vi "Auto Drive XY Right Automatic.vi"(0 "RobotDriveDevRef In":T2={"DevStatus"={"status"=FALSE, "code"=0, "source"=""}, "Motors[]"=[], "Square Inputs"=FALSE, "Max Output"=1.0}, 1 "Angle Offset":dbl, 3 "Movement":dbl=-1.0, 5 "Motor Output Range X":cluster{"output high":dbl, "output low":dbl}={"output high"=0.8, "output low"=-0.8}, 7 "PID Gains X":T1={"proportional gain (Kc)"=0.07, "integral time (Ti, min)"=0.0, "derivative time (Td, min)"=0.0}, 9 "Distance (in)":dbl=15.0 format="%#_13g", 11 "Time to Settle (ms)":u32=50, 12 "Min Time (ms)":u32=250, 13 "PID Gains Y":T1={"proportional gain (Kc)"=0.07, "integral time (Ti, min)"=0.0, "derivative time (Td, min)"=0.0}, 14 "Motor Output Range Y":cluster{"output high":dbl, "output low":dbl}={"output high"=0.7, "output low"=-0.7}, 15 "Max Time (ms)":u32=15000) -> (4 "RobotDriveDevRef Out":T2={"DevStatus"={"status"=FALSE, "code"=0, "source"=""}, "Motors[]"=[], "Square Inputs"=FALSE, "Max Output"=1.0})   [LabVIEW 2017]
uses:
  <vilib>/Rock Robotics/WPI/RobotDrive/WPI_RobotDriveDevRef.ctl
  <vilib>/Rock Robotics/WPI/MotorControl/WPI_MotorControlDeviceRef.ctl
  <vilib>/Rock Robotics/WPI/MotorControl/WPI_MotorControlType.ctl
  <vilib>/Rock Robotics/SystemInterfaces/DIO/FPGA_DIOPWMChannel.ctl
  <vilib>/Rock Robotics/WPI/PWM/WPI_PWMDeadband.ctl
  <vilib>/Rock Robotics/SystemInterfaces/DIO/FPGA_DIOChannel.ctl
  <vilib>/Rock Robotics/WPI/Solenoid/WPI_SolenoidValue.ctl
  Globals/Robot Global Data.vi
  <vilib>/addons/control/pid/pid.llb/PID (DBL).vi
  <vilib>/Rock Robotics/WPI/RobotDrive/WPI_RobotDriveArcadeDrive_Standard(NoSaturation).vi
  <vilib>/addons/control/pid/NI_PID_pid.lvlib
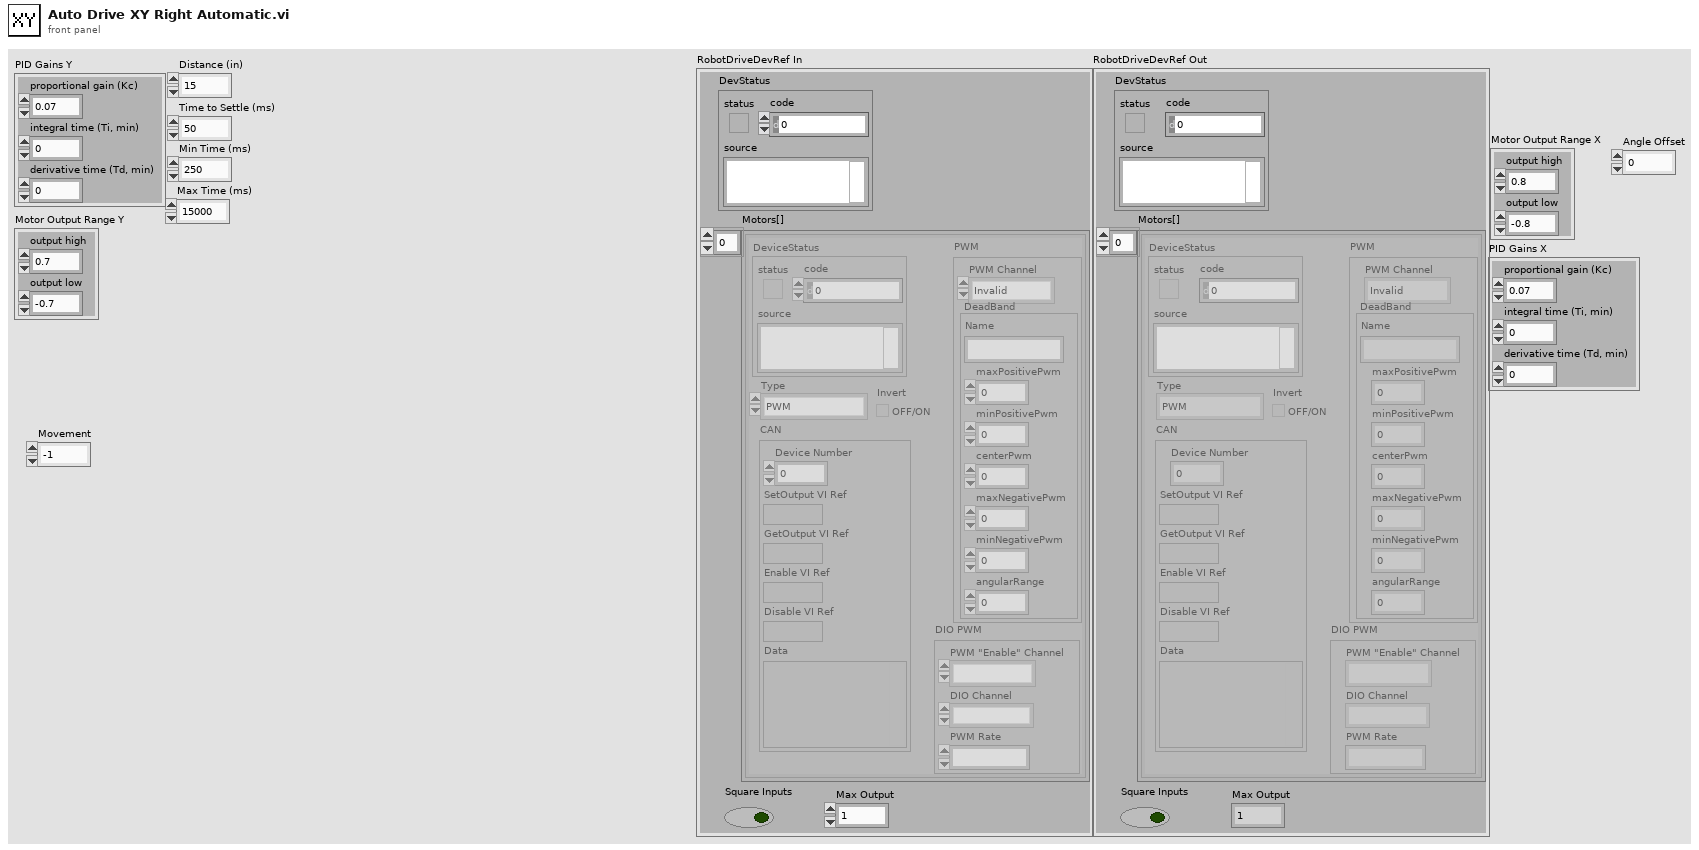
[diagram p1: front panel]
types:
  T1 = cluster{"proportional gain (Kc)":dbl, "integral time (Ti, min)":dbl, "derivative time (Td, min)":dbl}
  T2 = typedef "WPI_RobotDriveDevRef.ctl" = cluster{"DevStatus":errorcluster, "Motors[]":T3[], "Square Inputs":bool, "Max Output":dbl}
  T3 = typedef "WPI_MotorControlDeviceRef.ctl" = cluster{"DeviceStatus":errorcluster, "Type":T4, "PWM":cluster{"PWM Channel":T5, "DeadBand":T6}, "CAN":cluster{"Device Number":u8, "SetOutput VI Ref":variant, "GetOutput VI Ref":variant, "Enable VI Ref":variant, "Disable VI Ref":variant, "Data":variant}, "Invert":bool, "DIO PWM":cluster{"PWM \"Enable\" Channel":T5, "DIOChannel":T7, "PWM Rate":dbl}}
  T4 = typedef "WPI_MotorControlType.ctl" = enum16{"PWM", "CAN", "DIO PWM"}
  T5 = typedef "FPGA_DIOPWMChannel.ctl" = enum8{"PWM 0", "PWM 1", "PWM 2", "PWM 3", "PWM 4", "PWM 5", "PWM 6", "PWM 7", "PWM 8", "PWM 9", "PWM MXP 0", "PWM MXP 1", "PWM MXP 2", "PWM MXP 3", "PWM MXP 4", "PWM MXP 5", "PWM MXP 6", "PWM MXP 7", "PWM MXP 8", "PWM MXP 9", "Invalid"}
  T6 = typedef "WPI_PWMDeadband.ctl" = cluster{"Name":string, "maxPositivePwm":i32, "minPositivePwm":i32, "centerPwm":i32, "maxNegativePwm":i32, "minNegativePwm":i32, "angularRange":u16}
  T7 = typedef "FPGA_DIOChannel.ctl" = enum8{"DIO 0", "DIO 1", "DIO 2", "DIO 3", "DIO 4", "DIO 5", "DIO 6", "DIO 7", "DIO 8", "DIO 9", "DIO MXP 0", "DIO MXP 1", "DIO MXP 2", "DIO MXP 3", "DIO MXP 4", "DIO MXP 5", "DIO MXP 6", "DIO MXP 7", "DIO MXP 8", "DIO MXP 9", "DIO MXP 10", "DIO MXP 11", "DIO MXP 12", "DIO MXP 13", "DIO MXP 14", "DIO MXP 15", "SPI Port CS1", "SPI Port CS2", "SPI Port CS3", "SPI Port MISO", "SPI Port MOSI", "Invalid"}
  T8 = typedef "WPI_SolenoidValue.ctl" = enum16{"Off", "On", "Forward", "Reverse"}
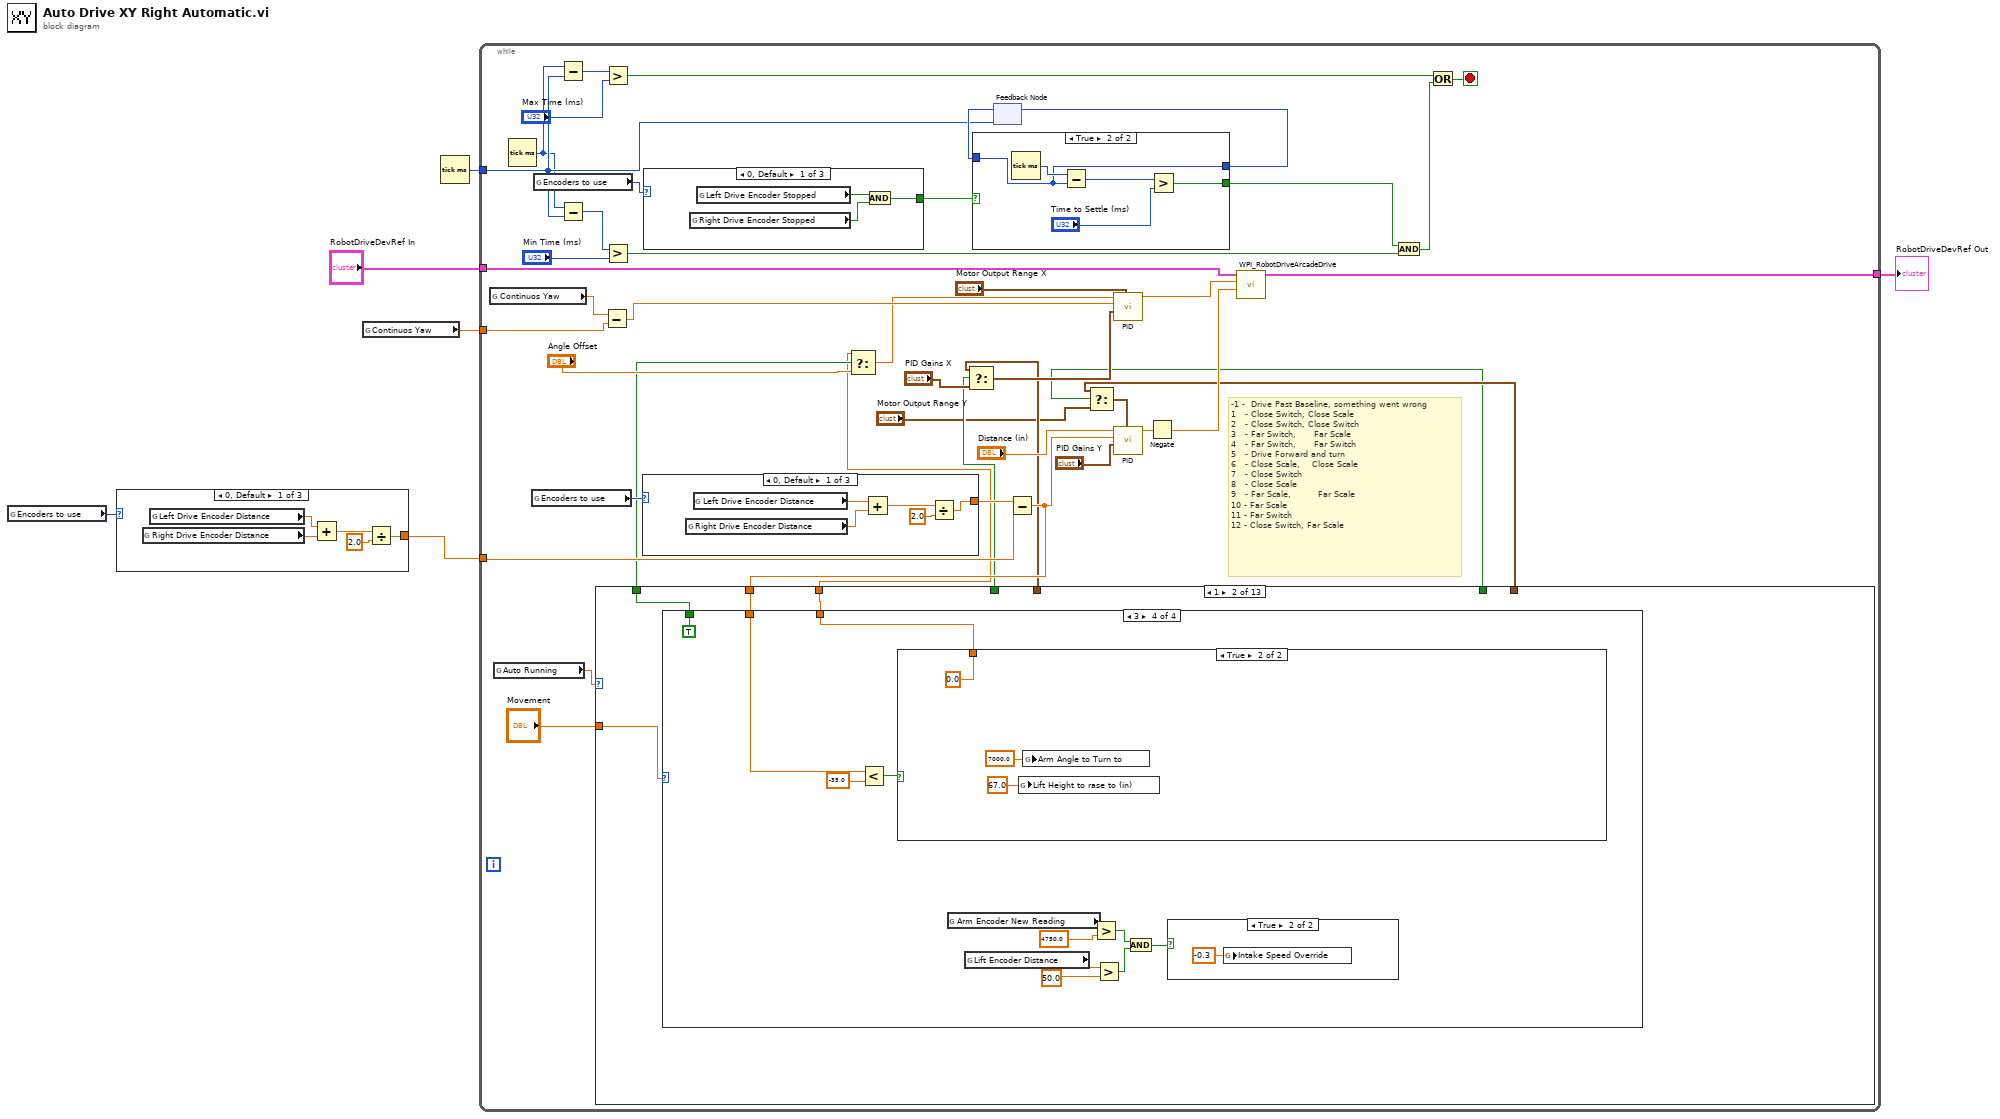
[diagram p0: block diagram]
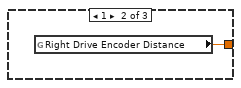
[diagram p2: hidden frame]
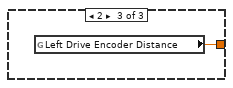
[diagram p3: hidden frame]
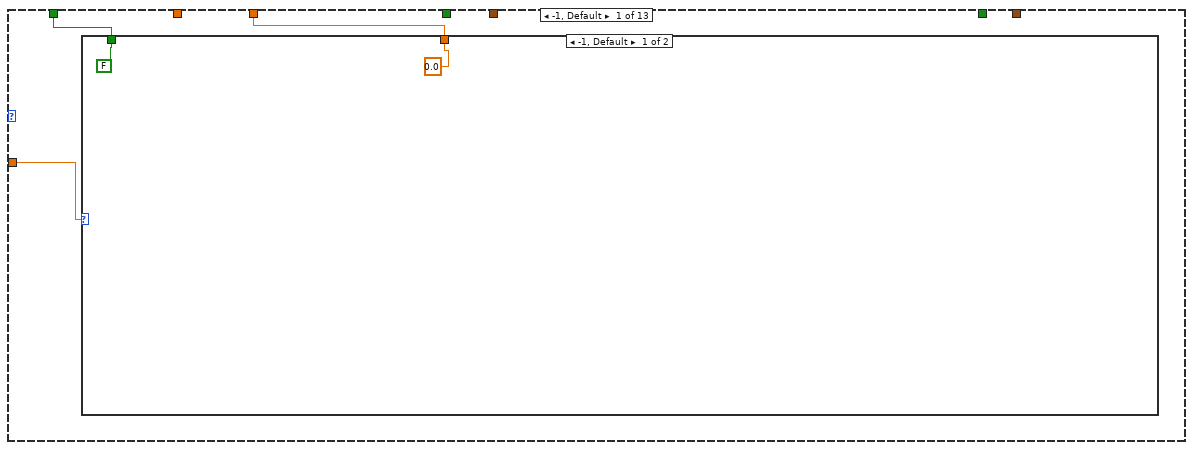
[diagram p4: hidden frame]
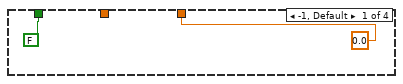
[diagram p6: hidden frame]
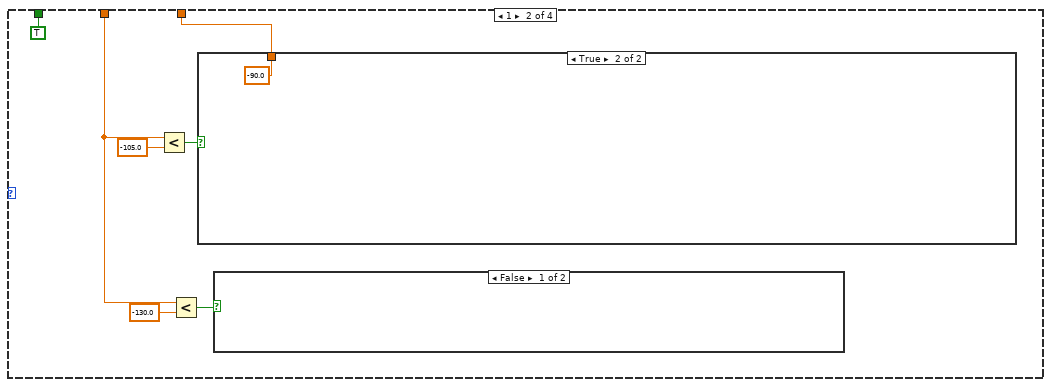
[diagram p7: hidden frame]
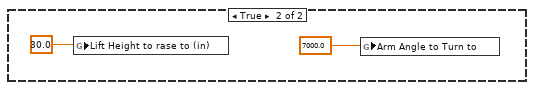
[diagram p8: hidden frame]
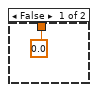
[diagram p9: hidden frame]
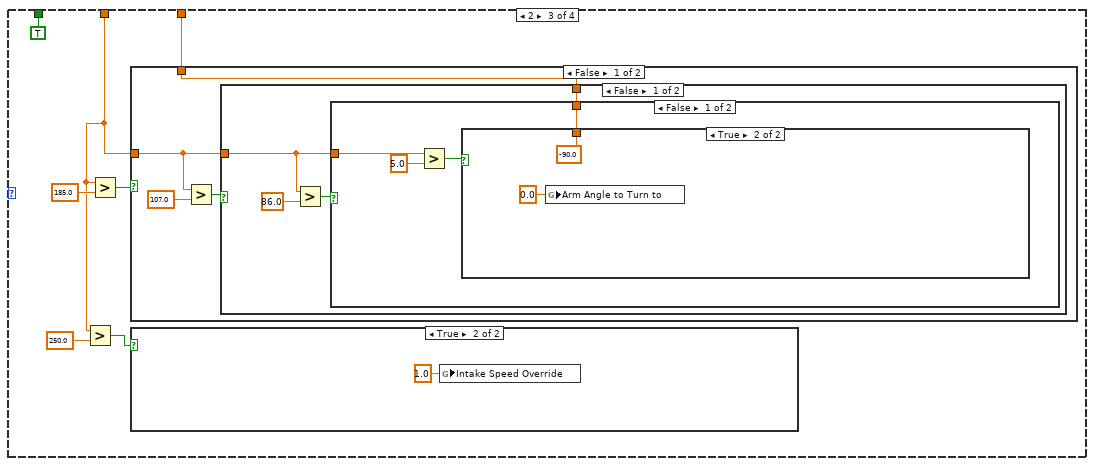
[diagram p10: hidden frame]
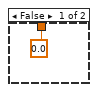
[diagram p11: hidden frame]
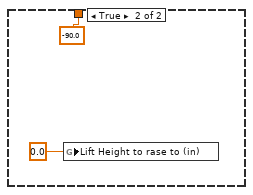
[diagram p12: hidden frame]
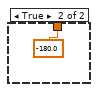
[diagram p13: hidden frame]
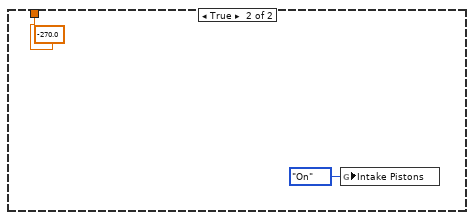
[diagram p14: hidden frame]
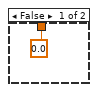
[diagram p17: hidden frame]
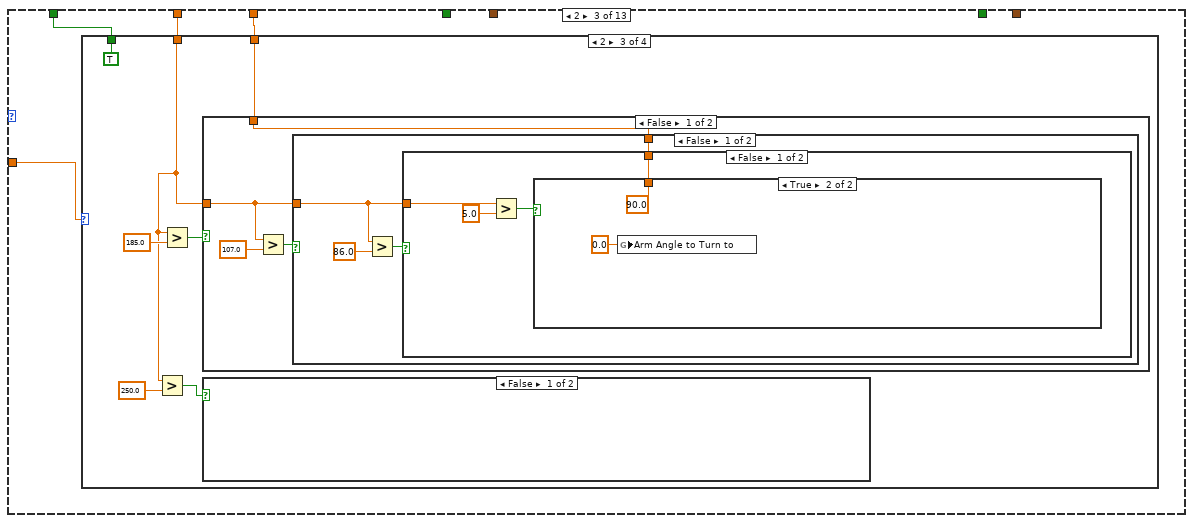
[diagram p18: hidden frame]
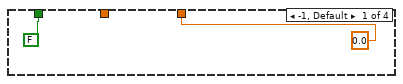
[diagram p19: hidden frame]
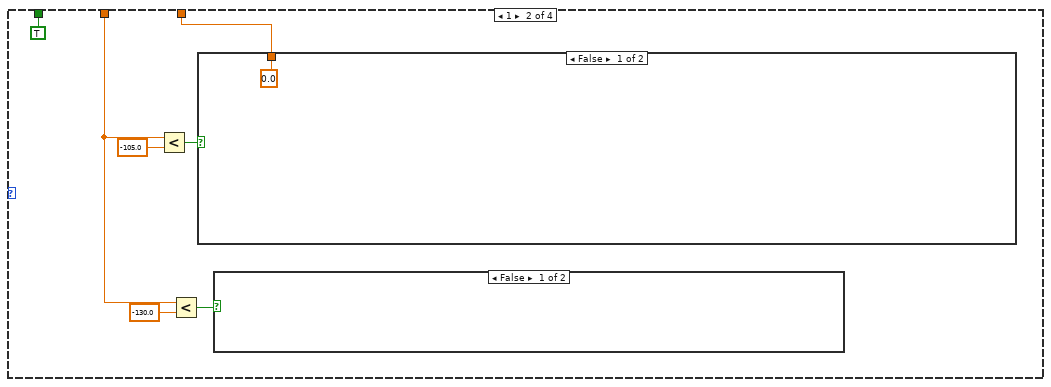
[diagram p20: hidden frame]
diagram:
  n1 = global read "Robot Global Data.vi" "Encoders to use"() -> (w2:u16)
  n2 = case shown="0, Default" w2 {
    tunnel: [w7 w12 w13] -> w6
    frame 0, Default {
      n3 = global read "Robot Global Data.vi" "Right Drive Encoder Distance"() -> (w10:dbl)
      n4 = global read "Robot Global Data.vi" "Left Drive Encoder Distance"() -> (w11:dbl)
      n5 = Add(x=w11, y=w10) -> (x+y=w9:dbl)
      n6 = Divide(x=w9, y=2.0) -> (x/y=w7:dbl)
    }
    frame 1 {
      n7 = global read "Robot Global Data.vi" "Right Drive Encoder Distance"() -> (w12:dbl)
    }
    frame 2 {
      n8 = global read "Robot Global Data.vi" "Left Drive Encoder Distance"() -> (w13:dbl)
    }
  }
  n9 = global read "Robot Global Data.vi" "Continuos Yaw"() -> (w1:dbl)
  n10 = Tick Count (ms)() -> (millisecond timer value=w5:u32)
  n11 = while {
    tunnel: "RobotDriveDevRef In" -> [w55]
    tunnel: w6 -> [w50]
    tunnel: w5 -> [w39]
    tunnel: [w49] -> w4
    tunnel: w1 -> [w30]
    stop <- w42 stop-if-true
    # "-1 -  Drive Past Baseline, something went wrong\n1   - Close Switch, Close Scale\n2   - Close Switch, Close Switch\n3   - Far Switch,      Far Scale\n4   - Far Switch,      Far Switch\n5   - Drive Forward and turn\n6   - Close Scale,    Close Scale\n7   - Close Switch\n8   - Close Scale\n9   - Far Scale,         Far Scale\n10 - Far Scale\n11 - Far Switch\n12 - Close Switch, Far Scale"
    n12 = global read "Robot Global Data.vi" "Continuos Yaw"() -> (w31:dbl)
    n13 = global read "Robot Global Data.vi" "Auto Running"() -> (w23:dbl)
    n14 = Tick Count (ms)() -> (millisecond timer value=w38:u32)
    n15 = global read "Robot Global Data.vi" "Encoders to use"() -> (w37:u16)
    n16 = global read "Robot Global Data.vi" "Encoders to use"() -> (w35:u16)
    n17 = Subtract(x=w38, y=w39) -> (x-y=w43:u32)
    n18 = Subtract(x=w38, y=w39) -> (x-y=w48:u32)
    n19 = Subtract(x=w31, y=w30) -> (x-y=w29:dbl)
    n20 = Greater?(x=w43, y="Max Time (ms)") -> (0:w40:bool)
    n21 = Greater?(x=w48, y="Min Time (ms)") -> (0:w45:bool)
    n22 = case shown="0, Default" w37 {
      tunnel: [w738 w743 w744] -> w36
      frame 0, Default {
        n23 = global read "Robot Global Data.vi" "Right Drive Encoder Distance"() -> (w741:dbl)
        n24 = global read "Robot Global Data.vi" "Left Drive Encoder Distance"() -> (w742:dbl)
        n25 = Add(x=w742, y=w741) -> (x+y=w740:dbl)
        n26 = Divide(x=w740, y=2.0) -> (x/y=w738:dbl)
      }
      frame 1 {
        n27 = global read "Robot Global Data.vi" "Right Drive Encoder Distance"() -> (w743:dbl)
      }
      frame 2 {
        n28 = global read "Robot Global Data.vi" "Left Drive Encoder Distance"() -> (w744:dbl)
      }
    }
    n29 = case shown="0, Default" w35 {
      tunnel: [w735 w736 w737] -> w34
      frame 0, Default {
        n30 = global read "Robot Global Data.vi" "Right Drive Encoder Stopped"() -> (w733:bool)
        n31 = global read "Robot Global Data.vi" "Left Drive Encoder Stopped"() -> (w734:bool)
        n32 = And(x=w734, y=w733) -> (x .and. y?=w735:bool)
      }
      frame 1 {
        n33 = global read "Robot Global Data.vi" "Right Drive Encoder Stopped"() -> (w736:bool)
      }
      frame 2 {
        n34 = global read "Robot Global Data.vi" "Left Drive Encoder Stopped"() -> (w737:bool)
      }
    }
    n35 = feedback #1(w39) -> (w51:u32)
    n36 = case shown="True" w34 {
      tunnel: w51 -> [_ w750]
      tunnel: [w746 w750] -> w52
      tunnel: [FALSE w747] -> w46
      frame False {
        n37 = Tick Count (ms)() -> (millisecond timer value=w746:u32)
      }
      frame True {
        n38 = Tick Count (ms)() -> (millisecond timer value=w751:u32)
        n39 = Subtract(x=w751, y=w750) -> (x-y=w749:u32)
        n40 = Greater?(x=w749, y="Time to Settle (ms)") -> (0:w747:bool)
      }
    }
    n41 = feedback-in #1(w52) -> ()
    n42 = Subtract(x=w36, y=w50) -> (x-y=w27:dbl)
    n43 = case shown="1" w23 {
      tunnel: "Movement" -> [w60 w66 w128 w175 w233 w281 w298 w397 w447 w502 w575 w614 w664]
      tunnel: w27 -> [_ w63 w125 w172 w230 w278 w295 w394 w444 w499 w572 w611 w661]
      tunnel: [w59 w65 w127 w174 w232 w280 w297 w396 w446 w501 w574 w613 w663] -> w24
      tunnel: [w58 w64 w126 w173 w231 w279 w296 w395 w445 w500 w573 w612 w662] -> w22
      tunnel: [_ _ _ _ _ _ w294 _ w443 w497 w571 _ _] -> w19
      tunnel: [_ _ _ _ _ _ w293 _ w442 w498 w570 _ _] -> w18
      tunnel: [_ _ _ _ _ _ w292 _ w440 w495 _ _ w659] -> w15
      tunnel: [_ _ _ _ _ _ w291 _ w441 w496 _ _ w660] -> w14
      frame -1, Default {
        n44 = case shown="-1, Default" w60 {
          tunnel: [FALSE _] -> w59
          tunnel: [0.0 _] -> w58
          frame -1, Default {
          }
          frame 1 {
          }
        }
      }
      frame 1 {
        n45 = case shown="3" w66 {
          tunnel: [FALSE TRUE TRUE TRUE] -> w65
          tunnel: [0.0 w72 w86 w116] -> w64
          tunnel: w63 -> [_ w70 w80 w115]
          frame -1, Default {
          }
          frame 1 {
            n46 = Less?(x=w70, y=-105.0) -> (x < y?=w74:bool)
            n47 = Less?(x=w70, y=-130.0) -> (x < y?=w69:bool)
            n48 = case shown="True" w74 {
              tunnel: [0.0 -90.0] -> w72
              frame False {
              }
              frame True {
              }
            }
            n49 = case shown="False" w69 {
              frame False {
              }
              frame True {
                n50 = global write "Robot Global Data.vi" "Lift Height to rase to (in)"(30.0 ("Auto Running")) -> ()
                n51 = global write "Robot Global Data.vi" "Arm Angle to Turn to"(7000.0 ("Auto Running")) -> ()
              }
            }
          }
          frame 2 {
            n52 = Greater?(x=w80, y=250.0) -> (0:w83:bool)
            n53 = Greater?(x=w80, y=185.0) -> (0:w81:bool)
            n54 = case shown="False" w81 {
              tunnel: [w90 -270.0] -> w86
              tunnel: w80 -> [w87 _]
              frame False {
                n55 = Greater?(x=w87, y=107.0) -> (0:w88:bool)
                n56 = case shown="False" w88 {
                  tunnel: [w94 -180.0] -> w90
                  tunnel: w87 -> [w91 _]
                  frame False {
                    n57 = Greater?(x=w91, y=86.0) -> (0:w92:bool)
                    n58 = case shown="False" w92 {
                      tunnel: w91 -> [w97 _]
                      tunnel: [w95 -90.0] -> w94
                      frame False {
                        n59 = Greater?(x=w97, y=5.0) -> (0:w98:bool)
                        n60 = case shown="True" w98 {
                          tunnel: [0.0 -90.0] -> w95
                          frame False {
                          }
                          frame True {
                            n61 = global write "Robot Global Data.vi" "Arm Angle to Turn to"(0.0 ("Arm Angle to Turn to")) -> ()
                          }
                        }
                      }
                      frame True {
                        n62 = global write "Robot Global Data.vi" "Lift Height to rase to (in)"(0.0 ("Arm Angle to Turn to")) -> ()
                      }
                    }
                  }
                  frame True {
                  }
                }
              }
              frame True {
                n63 = global write "Robot Global Data.vi" "Intake Pistons"(WPI_SolenoidValue."On" ("Intake Pistons")) -> ()
              }
            }
            n64 = case shown="True" w83 {
              frame False {
              }
              frame True {
                n65 = global write "Robot Global Data.vi" "Intake Speed Override"(1.0 ("Arm Angle to Turn to")) -> ()
              }
            }
          }
          frame 3 {
            n66 = Less?(x=w115, y=-35.0) -> (x < y?=w119:bool)
            n67 = case shown="True" w119 {
              tunnel: [0.0 0.0] -> w116
              frame False {
              }
              frame True {
                n68 = global write "Robot Global Data.vi" "Lift Height to rase to (in)"(67.0 ("Arm Angle to Turn to")) -> ()
                n69 = global write "Robot Global Data.vi" "Arm Angle to Turn to"(7000.0 ("Arm Angle to Turn to")) -> ()
              }
            }
            n70 = global read "Robot Global Data.vi" "Arm Encoder New Reading"() -> (w113:dbl)
            n71 = global read "Robot Global Data.vi" "Lift Encoder Distance"() -> (w114:dbl)
            n72 = Greater?(x=w113, y=4750.0 ("Arm Angle to Turn to")) -> (0:w110:bool)
            n73 = Greater?(x=w114, y=50.0 ("Arm Angle to Turn to")) -> (0:w109:bool)
            n74 = And(x=w110, y=w109) -> (x .and. y?=w108:bool)
            n75 = case shown="True" w108 {
              frame False {
              }
              frame True {
                n76 = global write "Robot Global Data.vi" "Intake Speed Override"(-0.3 ("Arm Angle to Turn to")) -> ()
              }
            }
          }
        }
      }
      frame 2 {
        n77 = case shown="2" w128 {
          tunnel: [FALSE TRUE TRUE TRUE] -> w127
          tunnel: [0.0 w134 w142 0.0] -> w126
          tunnel: w125 -> [_ w132 w143 _]
          frame -1, Default {
          }
          frame 1 {
            n78 = Less?(x=w132, y=-105.0) -> (x < y?=w136:bool)
            n79 = Less?(x=w132, y=-130.0) -> (x < y?=w131:bool)
            n80 = case shown="False" w136 {
              tunnel: [0.0 90.0] -> w134
              frame False {
              }
              frame True {
              }
            }
            n81 = case shown="False" w131 {
              frame False {
              }
              frame True {
                n82 = global write "Robot Global Data.vi" "Lift Height to rase to (in)"(30.0 ("Auto Running")) -> ()
                n83 = global write "Robot Global Data.vi" "Arm Angle to Turn to"(7000.0 ("Auto Running")) -> ()
              }
            }
          }
          frame 2 {
            n84 = Greater?(x=w143, y=250.0) -> (0:w146:bool)
            n85 = Greater?(x=w143, y=185.0) -> (0:w144:bool)
            n86 = case shown="False" w144 {
              tunnel: [w152 270.0] -> w142
              tunnel: w143 -> [w149 _]
              frame False {
                n87 = Greater?(x=w149, y=107.0) -> (0:w150:bool)
                n88 = case shown="False" w150 {
                  tunnel: [w156 180.0] -> w152
                  tunnel: w149 -> [w153 _]
                  frame False {
                    n89 = Greater?(x=w153, y=86.0) -> (0:w154:bool)
                    n90 = case shown="False" w154 {
                      tunnel: w153 -> [w159 _]
                      tunnel: [w157 90.0] -> w156
                      frame False {
                        n91 = Greater?(x=w159, y=5.0) -> (0:w160:bool)
                        n92 = case shown="True" w160 {
                          tunnel: [0.0 90.0] -> w157
                          frame False {
                          }
                          frame True {
                            n93 = global write "Robot Global Data.vi" "Arm Angle to Turn to"(0.0 ("Arm Angle to Turn to")) -> ()
                          }
                        }
                      }
                      frame True {
                        n94 = global write "Robot Global Data.vi" "Lift Height to rase to (in)"(0.0 ("Arm Angle to Turn to")) -> ()
                      }
                    }
                  }
                  frame True {
                  }
                }
              }
              frame True {
                n95 = global write "Robot Global Data.vi" "Intake Pistons"(WPI_SolenoidValue."On" ("Intake Pistons")) -> ()
              }
            }
            n96 = case shown="False" w146 {
              frame False {
              }
              frame True {
                n97 = global write "Robot Global Data.vi" "Intake Speed Override"(1.0 ("Arm Angle to Turn to")) -> ()
              }
            }
          }
          frame 3 {
          }
        }
      }
      frame 3 {
        n98 = case shown="1" w175 {
          tunnel: [FALSE TRUE TRUE TRUE] -> w174
          tunnel: [0.0 w181 w198 0.0] -> w173
          tunnel: w172 -> [_ w178 w192 w220]
          frame -1, Default {
          }
          frame 1 {
            n99 = Less?(x=w178, y=-300.0) -> (x < y?=w179:bool)
            n100 = case shown="False" w179 {
              tunnel: [w184 270.0] -> w181
              tunnel: w178 -> [w183 _]
              frame False {
                n101 = Less?(x=w183, y=-100.0) -> (x < y?=w186:bool)
                n102 = case shown="True" w186 {
                  tunnel: [0.0 90.0] -> w184
                  frame False {
                  }
                  frame True {
                  }
                }
              }
              frame True {
                n103 = global write "Robot Global Data.vi" "Lift Height to rase to (in)"(20.0 ("Arm Angle to Turn to")) -> ()
                n104 = global write "Robot Global Data.vi" "Arm Angle to Turn to"(7000.0 ("Arm Angle to Turn to")) -> ()
              }
            }
          }
          frame 2 {
            n105 = Greater?(x=w192, y=70.0) -> (0:w195:bool)
            n106 = case shown="True" w195 {
              frame False {
              }
              frame True {
                n107 = global write "Robot Global Data.vi" "Intake Speed Override"(1.0 ("Arm Angle to Turn to")) -> ()
                n108 = global write "Robot Global Data.vi" "Intake Pistons"(WPI_SolenoidValue."On" ("Intake Pistons")) -> ()
              }
            }
            n109 = Greater?(x=w192, y=100.0) -> (0:w193:bool)
            n110 = case shown="False" w193 {
              tunnel: [w202 -270.0] -> w198
              tunnel: w192 -> [w199 _]
              frame False {
                n111 = Greater?(x=w199, y=50.0) -> (0:w200:bool)
                n112 = case shown="False" w200 {
                  tunnel: [w206 -180.0] -> w202
                  tunnel: w199 -> [w205 _]
                  frame False {
                    n113 = Greater?(x=w205, y=25.0) -> (0:w203:bool)
                    n114 = case shown="False" w203 {
                      tunnel: w205 -> [w209 _]
                      tunnel: [w207 -90.0] -> w206
                      frame False {
                        n115 = Greater?(x=w209, y=8.5) -> (0:w210:bool)
                        n116 = case shown="True" w210 {
                          tunnel: [0.0 -90.0] -> w207
                          frame False {
                          }
                          frame True {
                            n117 = global write "Robot Global Data.vi" "Arm Angle to Turn to"(0.0 ("Arm Angle to Turn to")) -> ()
                          }
                        }
                      }
                      frame True {
                        n118 = global write "Robot Global Data.vi" "Lift Height to rase to (in)"(0.0 ("Arm Angle to Turn to")) -> ()
                      }
                    }
                  }
                  frame True {
                  }
                }
              }
              frame True {
              }
            }
          }
          frame 3 {
            n119 = Less?(x=w220, y=-40.0) -> (x < y?=w222:bool)
            n120 = Less?(x=w220, y=-60.0) -> (x < y?=w224:bool)
            n121 = case shown="True" w222 {
              frame False {
              }
              frame True {
                n122 = global write "Robot Global Data.vi" "Lift Height to rase to (in)"(67.0 ("Arm Angle to Turn to")) -> ()
                n123 = global write "Robot Global Data.vi" "Arm Angle to Turn to"(7000.0 ("Arm Angle to Turn to")) -> ()
              }
            }
            n124 = case shown="True" w224 {
              frame False {
              }
              frame True {
                n125 = global write "Robot Global Data.vi" "Intake Speed Override"(-1.0 ("Arm Angle to Turn to")) -> ()
              }
            }
          }
        }
      }
      frame 4 {
        n126 = case shown="1" w233 {
          tunnel: [FALSE TRUE TRUE] -> w232
          tunnel: [0.0 w236 w251] -> w231
          tunnel: w230 -> [_ w237 w252]
          frame -1, Default {
          }
          frame 1 {
            n127 = Less?(x=w237, y=-300.0) -> (x < y?=w239:bool)
            n128 = case shown="False" w239 {
              tunnel: [w242 270.0] -> w236
              tunnel: w237 -> [w241 _]
              frame False {
                n129 = Less?(x=w241, y=-100.0) -> (x < y?=w244:bool)
                n130 = case shown="True" w244 {
                  tunnel: [0.0 90.0] -> w242
                  frame False {
                  }
                  frame True {
                  }
                }
              }
              frame True {
                n131 = global write "Robot Global Data.vi" "Lift Height to rase to (in)"(20.0 ("Arm Angle to Turn to")) -> ()
                n132 = global write "Robot Global Data.vi" "Arm Angle to Turn to"(7000.0 ("Arm Angle to Turn to")) -> ()
              }
            }
          }
          frame 2 {
            n133 = Greater?(x=w252, y=70.0) -> (0:w255:bool)
            n134 = case shown="True" w255 {
              frame False {
              }
              frame True {
                n135 = global write "Robot Global Data.vi" "Intake Speed Override"(1.0 ("Arm Angle to Turn to")) -> ()
                n136 = global write "Robot Global Data.vi" "Intake Pistons"(WPI_SolenoidValue."On" ("Intake Pistons")) -> ()
              }
            }
            n137 = Greater?(x=w252, y=100.0) -> (0:w253:bool)
            n138 = case shown="False" w253 {
              tunnel: [w260 -270.0] -> w251
              tunnel: w252 -> [w257 _]
              frame False {
                n139 = Greater?(x=w257, y=50.0) -> (0:w258:bool)
                n140 = case shown="False" w258 {
                  tunnel: [w264 -180.0] -> w260
                  tunnel: w257 -> [w263 _]
                  frame False {
                    n141 = Greater?(x=w263, y=25.0) -> (0:w261:bool)
                    n142 = case shown="False" w261 {
                      tunnel: w263 -> [w267 _]
                      tunnel: [w265 -90.0] -> w264
                      frame False {
                        n143 = Greater?(x=w267, y=8.5) -> (0:w268:bool)
                        n144 = case shown="True" w268 {
                          tunnel: [0.0 -90.0] -> w265
                          frame False {
                          }
                          frame True {
                            n145 = global write "Robot Global Data.vi" "Arm Angle to Turn to"(0.0 ("Arm Angle to Turn to")) -> ()
                          }
                        }
                      }
                      frame True {
                        n146 = global write "Robot Global Data.vi" "Lift Height to rase to (in)"(0.0 ("Arm Angle to Turn to")) -> ()
                      }
                    }
                  }
                  frame True {
                  }
                }
              }
              frame True {
              }
            }
          }
        }
      }
      frame 5 {
        n147 = case shown="1" w281 {
          tunnel: [FALSE TRUE] -> w280
          tunnel: [0.0 w287] -> w279
          tunnel: w278 -> [_ w286]
          frame -1, Default {
          }
          frame 1 {
            n148 = Less?(x=w286, y=-174.0) -> (x < y?=w285:bool)
            n149 = case shown="True" w285 {
              tunnel: [0.0 90.0] -> w287
              frame False {
              }
              frame True {
              }
            }
          }
        }
      }
      frame 6 {
        n150 = case shown="3" w298 {
          tunnel: [FALSE TRUE TRUE TRUE] -> w297
          tunnel: [0.0 w326 w349 w372] -> w296
          tunnel: w295 -> [_ w301 w346 w376]
          tunnel: [_ w317 _ w375] -> w294
          tunnel: [_ w316 _ w374] -> w293
          tunnel: [_ w313 _ _] -> w292
          tunnel: [_ w314 _ _] -> w291
          frame -1, Default {
          }
          frame 1 {
            n151 = global read "Robot Global Data.vi" "Arm Encoder New Reading"() -> (w310:dbl)
            n152 = global read "Robot Global Data.vi" "Lift Encoder Distance"() -> (w311:dbl)
            n153 = Less?(x=w301, y=-250.0) -> (x < y?=w321:bool)
            n154 = case shown="True" w321 {
              frame False {
              }
              frame True {
                n155 = global write "Robot Global Data.vi" "Arm Angle to Turn to"(7000.0 ("Arm Angle to Turn to")) -> ()
              }
            }
            n156 = Greater?(x=w310, y=4500.0 ("Arm Angle to Turn to")) -> (0:w307:bool)
            n157 = Greater?(x=w311, y=45.0 ("Arm Angle to Turn to")) -> (0:w306:bool)
            n158 = And(x=w307, y=w306) -> (x .and. y?=w302:bool)
            n159 = Less?(x=w301, y=-260.0) -> (x < y?=w303:bool)
            n160 = And(x=w302, y=w303) -> (x .and. y?=w304:bool)
            n161 = Less?(x=w301, y=-260.0) -> (x < y?=w318:bool)
            n162 = case shown="True" w304 {
              frame False {
              }
              frame True {
                n163 = global write "Robot Global Data.vi" "Intake Speed Override"(-0.5 ("Arm Angle to Turn to")) -> ()
              }
            }
            n164 = case shown="True" w318 {
              tunnel: [FALSE TRUE] -> w317
              tunnel: [T1 {"proportional gain (Kc)"=0.0, "integral time (Ti, min)"=0.0, "derivative time (Td, min)"=0.0} ("t") T1 {"proportional gain (Kc)"=0.035, "integral time (Ti, min)"=0.0, "derivative time (Td, min)"=0.0} ("t")] -> w316
              frame False {
              }
              frame True {
              }
            }
            n165 = Less?(x=w301, y=-250.0) -> (x < y?=w325:bool)
            n166 = case shown="False" w325 {
              tunnel: [w342 0.0] -> w326
              tunnel: w301 -> [w339 _]
              frame False {
                n167 = Less?(x=w339, y=-120.0) -> (x < y?=w341:bool)
                n168 = case shown="True" w341 {
                  tunnel: [0.0 -90.0] -> w342
                  frame False {
                  }
                  frame True {
                  }
                }
              }
              frame True {
              }
            }
            n169 = Less?(x=w301, y=-180.0) -> (x < y?=w322:bool)
            n170 = case shown="True" w322 {
              frame False {
              }
              frame True {
                n171 = global write "Robot Global Data.vi" "Lift Height to rase to (in)"(67.0 ("Arm Angle to Turn to")) -> ()
              }
            }
            n172 = Less?(x=w301, y=-250.0) -> (x < y?=w312:bool)
            n173 = case shown="True" w312 {
              tunnel: [FALSE TRUE] -> w314
              tunnel: [cluster{"output high":dbl, "output low":dbl} {"output high"=0.0, "output low"=0.0} ("s? t:f") cluster{"output high":dbl, "output low":dbl} {"output high"=0.6, "output low"=-0.5} ("s? t:f")] -> w313
              frame False {
              }
              frame True {
              }
            }
          }
          frame 2 {
            n174 = global write "Robot Global Data.vi" "Lift Height to rase to (in)"(0.0 ("Arm Angle to Turn to")) -> ()
            n175 = global write "Robot Global Data.vi" "Arm Angle to Turn to"(0.0 ("Arm Angle to Turn to")) -> ()
            n176 = Greater?(x=w346, y=30.0) -> (0:w351:bool)
            n177 = Greater?(x=w346, y=30.0) -> (0:w347:bool)
            n178 = case shown="False" w351 {
              tunnel: [w360 0.0] -> w349
              tunnel: w346 -> [w357 _]
              frame False {
                n179 = Greater?(x=w357, y=10.0) -> (0:w359:bool)
                n180 = case shown="True" w359 {
                  tunnel: [0.0 20.0] -> w360
                  frame False {
                  }
                  frame True {
                  }
                }
              }
              frame True {
              }
            }
            n181 = case shown="True" w347 {
              frame False {
              }
              frame True {
                n182 = global write "Robot Global Data.vi" "Intake Speed Override"(1.0 ("Arm Angle to Turn to")) -> ()
                n183 = global write "Robot Global Data.vi" "Intake Pistons"(WPI_SolenoidValue."On" ("Intake Pistons")) -> ()
              }
            }
          }
          frame 3 {
            n184 = Less?(x=w376, y=-30.0) -> (x < y?=w378:bool)
            n185 = case shown="False" w378 {
              tunnel: [w387 0.0] -> w372
              tunnel: w376 -> [w384 _]
              frame False {
                n186 = Less?(x=w384, y=0.0) -> (x < y?=w386:bool)
                n187 = case shown="True" w386 {
                  tunnel: [0.0 20.0] -> w387
                  frame False {
                  }
                  frame True {
                  }
                }
              }
              frame True {
              }
            }
            n188 = global read "Robot Global Data.vi" "Arm Encoder New Reading"() -> (w369:dbl)
            n189 = global read "Robot Global Data.vi" "Lift Encoder Distance"() -> (w370:dbl)
            n190 = Less?(x=w372, y=-40.0) -> (x < y?=w371:bool)
            n191 = case shown="False" w371 {
              tunnel: [_ TRUE] -> w375
              tunnel: [_ T1 {"proportional gain (Kc)"=0.0, "integral time (Ti, min)"=0.0, "derivative time (Td, min)"=0.0} ("t")] -> w374
              frame False {
              }
              frame True {
              }
            }
            n192 = Greater?(x=w369, y=5500.0 ("Arm Angle to Turn to")) -> (0:w366:bool)
            n193 = Greater?(x=w370, y=50.0 ("Arm Angle to Turn to")) -> (0:w365:bool)
            n194 = And(x=w366, y=w365) -> (x .and. y?=w364:bool)
            n195 = Less?(x=w376, y=-30.0) -> (x < y?=w380:bool)
            n196 = case shown="True" w364 {
              frame False {
              }
              frame True {
                n197 = global write "Robot Global Data.vi" "Intake Speed Override"(-0.4 ("Arm Angle to Turn to")) -> ()
              }
            }
            n198 = case shown="True" w380 {
              frame False {
              }
              frame True {
                n199 = global write "Robot Global Data.vi" "Lift Height to rase to (in)"(67.0 ("Arm Angle to Turn to")) -> ()
                n200 = global write "Robot Global Data.vi" "Arm Angle to Turn to"(7000.0 ("Arm Angle to Turn to")) -> ()
              }
            }
          }
        }
      }
      frame 7 {
        n201 = case shown="2" w397 {
          tunnel: [FALSE TRUE TRUE] -> w396
          tunnel: [0.0 w403 w413] -> w395
          tunnel: w394 -> [_ w401 w412]
          frame -1, Default {
          }
          frame 1 {
            n202 = Less?(x=w401, y=-105.0) -> (x < y?=w405:bool)
            n203 = Less?(x=w401, y=-130.0) -> (x < y?=w400:bool)
            n204 = case shown="True" w405 {
              tunnel: [0.0 90.0] -> w403
              frame False {
              }
              frame True {
              }
            }
            n205 = case shown="True" w400 {
              frame False {
              }
              frame True {
                n206 = global write "Robot Global Data.vi" "Lift Height to rase to (in)"(30.0 ("Auto Running")) -> ()
                n207 = global write "Robot Global Data.vi" "Arm Angle to Turn to"(7000.0 ("Auto Running")) -> ()
              }
            }
          }
          frame 2 {
            n208 = Greater?(x=w412, y=250.0) -> (0:w416:bool)
            n209 = Greater?(x=w412, y=185.0) -> (0:w414:bool)
            n210 = case shown="False" w414 {
              tunnel: [w421 270.0] -> w413
              tunnel: w412 -> [w418 _]
              frame False {
                n211 = Greater?(x=w418, y=107.0) -> (0:w419:bool)
                n212 = case shown="False" w419 {
                  tunnel: [w425 180.0] -> w421
                  tunnel: w418 -> [w422 _]
                  frame False {
                    n213 = Greater?(x=w422, y=86.0) -> (0:w423:bool)
                    n214 = case shown="False" w423 {
                      tunnel: w422 -> [w428 _]
                      tunnel: [w426 90.0] -> w425
                      frame False {
                        n215 = Greater?(x=w428, y=5.0) -> (0:w429:bool)
                        n216 = case shown="True" w429 {
                          tunnel: [0.0 90.0] -> w426
                          frame False {
                          }
                          frame True {
                            n217 = global write "Robot Global Data.vi" "Arm Angle to Turn to"(0.0 ("Arm Angle to Turn to")) -> ()
                          }
                        }
                      }
                      frame True {
                        n218 = global write "Robot Global Data.vi" "Lift Height to rase to (in)"(0.0 ("Arm Angle to Turn to")) -> ()
                      }
                    }
                  }
                  frame True {
                  }
                }
              }
              frame True {
                n219 = global write "Robot Global Data.vi" "Intake Pistons"(WPI_SolenoidValue."On" ("Intake Pistons")) -> ()
              }
            }
            n220 = case shown="True" w416 {
              frame False {
              }
              frame True {
                n221 = global write "Robot Global Data.vi" "Intake Speed Override"(1.0 ("Arm Angle to Turn to")) -> ()
                n222 = global write "Robot Global Data.vi" "Intake Pistons"(WPI_SolenoidValue."On" ("Intake Pistons")) -> ()
              }
            }
          }
        }
      }
      frame 8 {
        n223 = case shown="1" w447 {
          tunnel: [FALSE TRUE] -> w446
          tunnel: [0.0 w454] -> w445
          tunnel: w444 -> [_ w455]
          tunnel: [_ w453] -> w443
          tunnel: [_ w452] -> w442
          tunnel: [_ w451] -> w441
          tunnel: [_ w450] -> w440
          frame -1, Default {
          }
          frame 1 {
            n224 = global read "Robot Global Data.vi" "Arm Encoder New Reading"() -> (w465:dbl)
            n225 = global read "Robot Global Data.vi" "Lift Encoder Distance"() -> (w466:dbl)
            n226 = Less?(x=w455, y=-220.0) -> (x < y?=w472:bool)
            n227 = case shown="True" w472 {
              frame False {
              }
              frame True {
                n228 = global write "Robot Global Data.vi" "Arm Angle to Turn to"(7000.0 ("Arm Angle to Turn to")) -> ()
              }
            }
            n229 = Greater?(x=w465, y=4500.0 ("Arm Angle to Turn to")) -> (0:w462:bool)
            n230 = Greater?(x=w466, y=45.0 ("Arm Angle to Turn to")) -> (0:w461:bool)
            n231 = And(x=w462, y=w461) -> (x .and. y?=w457:bool)
            n232 = Less?(x=w455, y=-260.0) -> (x < y?=w458:bool)
            n233 = And(x=w457, y=w458) -> (x .and. y?=w459:bool)
            n234 = Less?(x=w455, y=-210.0) -> (x < y?=w469:bool)
            n235 = case shown="True" w459 {
              frame False {
              }
              frame True {
                n236 = global write "Robot Global Data.vi" "Intake Speed Override"(-0.5 ("Arm Angle to Turn to")) -> ()
              }
            }
            n237 = case shown="True" w469 {
              tunnel: [FALSE TRUE] -> w453
              tunnel: [T1 {"proportional gain (Kc)"=0.0, "integral time (Ti, min)"=0.0, "derivative time (Td, min)"=0.0} ("t") T1 {"proportional gain (Kc)"=0.035, "integral time (Ti, min)"=0.0, "derivative time (Td, min)"=0.0} ("t")] -> w452
              frame False {
              }
              frame True {
              }
            }
            n238 = Less?(x=w455, y=-160.0) -> (x < y?=w476:bool)
            n239 = case shown="False" w476 {
              tunnel: [w491 0.0] -> w454
              tunnel: w455 -> [w488 _]
              frame False {
                n240 = Less?(x=w488, y=-88.0) -> (x < y?=w490:bool)
                n241 = case shown="False" w490 {
                  tunnel: [0.0 90.0] -> w491
                  frame False {
                  }
                  frame True {
                  }
                }
              }
              frame True {
              }
            }
            n242 = Less?(x=w455, y=-190.0) -> (x < y?=w473:bool)
            n243 = case shown="True" w473 {
              frame False {
              }
              frame True {
                n244 = global write "Robot Global Data.vi" "Lift Height to rase to (in)"(67.0 ("Arm Angle to Turn to")) -> ()
              }
            }
            n245 = Less?(x=w455, y=-200.0) -> (x < y?=w467:bool)
            n246 = case shown="True" w467 {
              tunnel: [FALSE TRUE] -> w451
              tunnel: [cluster{"output high":dbl, "output low":dbl} {"output high"=0.0, "output low"=0.0} ("s? t:f") cluster{"output high":dbl, "output low":dbl} {"output high"=0.6, "output low"=-0.5} ("s? t:f")] -> w450
              frame False {
              }
              frame True {
              }
            }
          }
        }
      }
      frame 9 {
        n247 = case shown="1" w502 {
          tunnel: [FALSE TRUE FALSE _] -> w501
          tunnel: [0.0 w528 _ _] -> w500
          tunnel: w499 -> [_ w506 w544 w554]
          tunnel: [_ w523 _ _] -> w498
          tunnel: [_ w522 _ _] -> w497
          tunnel: [_ w507 _ _] -> w496
          tunnel: [_ w505 _ _] -> w495
          frame -1, Default {
          }
          frame 1 {
            n248 = global read "Robot Global Data.vi" "Arm Encoder New Reading"() -> (w520:dbl)
            n249 = global read "Robot Global Data.vi" "Lift Encoder Distance"() -> (w521:dbl)
            n250 = Greater?(x=w520, y=4500.0 ("Arm Angle to Turn to")) -> (0:w517:bool)
            n251 = Greater?(x=w521, y=55.0 ("Arm Angle to Turn to")) -> (0:w516:bool)
            n252 = And(x=w517, y=w516) -> (x .and. y?=w512:bool)
            n253 = Less?(x=w506, y=-395.0) -> (x < y?=w513:bool)
            n254 = Less?(x=w506, y=-350.0) -> (x < y?=w524:bool)
            n255 = And(x=w512, y=w513) -> (x .and. y?=w514:bool)
            n256 = Less?(x=w506, y=-285.0) -> (x < y?=w526:bool)
            n257 = case shown="True" w524 {
              tunnel: [_ T1 {"proportional gain (Kc)"=0.03, "integral time (Ti, min)"=0.0, "derivative time (Td, min)"=0.0} ("t")] -> w523
              tunnel: [_ TRUE] -> w522
              frame False {
              }
              frame True {
              }
            }
            n258 = case shown="True" w514 {
              frame False {
              }
              frame True {
                n259 = global write "Robot Global Data.vi" "Intake Speed Override"(-0.1 ("Arm Angle to Turn to")) -> ()
              }
            }
            n260 = case shown="False" w526 {
              tunnel: [w538 -15.0] -> w528
              tunnel: w506 -> [w537 _]
              frame False {
                n261 = Less?(x=w537, y=-115.0) -> (x < y?=w540:bool)
                n262 = case shown="True" w540 {
                  tunnel: [0.0 90.0] -> w538
                  frame False {
                  }
                  frame True {
                  }
                }
              }
              frame True {
              }
            }
            n263 = Less?(x=w506, y=-250.0) -> (x < y?=w510:bool)
            n264 = Less?(x=w506, y=-350.0) -> (x < y?=w508:bool)
            n265 = case shown="True" w510 {
              frame False {
              }
              frame True {
                n266 = global write "Robot Global Data.vi" "Lift Height to rase to (in)"(67.0 ("Arm Angle to Turn to")) -> ()
                n267 = global write "Robot Global Data.vi" "Arm Angle to Turn to"(7000.0 ("Arm Angle to Turn to")) -> ()
              }
            }
            n268 = case shown="True" w508 {
              tunnel: [_ TRUE] -> w507
              tunnel: [_ cluster{"output high":dbl, "output low":dbl} {"output high"=0.6, "output low"=-0.6} ("s? t:f")] -> w505
              frame False {
              }
              frame True {
              }
            }
          }
          frame 2 {
            n269 = Greater?(x=w544, y=30.0) -> (0:w548:bool)
            n270 = Greater?(x=w544, y=10.0) -> (0:w546:bool)
            n271 = case shown="True" w548 {
              frame False {
              }
              frame True {
                n272 = global write "Robot Global Data.vi" "Intake Speed Override"(1.0 ("Arm Angle to Turn to")) -> ()
              }
            }
            n273 = case shown="True" w546 {
              frame False {
              }
              frame True {
                n274 = global write "Robot Global Data.vi" "Lift Height to rase to (in)"(0.0 ("Arm Angle to Turn to")) -> ()
                n275 = global write "Robot Global Data.vi" "Arm Angle to Turn to"(0.0 ("Arm Angle to Turn to")) -> ()
              }
            }
            n276 = global write "Robot Global Data.vi" "Intake Pistons"(WPI_SolenoidValue."On" ("Intake Pistons")) -> ()
          }
          frame 3 {
            n277 = global read "Robot Global Data.vi" "Arm Encoder New Reading"() -> (w563:dbl)
            n278 = global read "Robot Global Data.vi" "Lift Encoder Distance"() -> (w564:dbl)
            n279 = Less?(x=w554, y=-10.0) -> (x < y?=w565:bool)
            n280 = Greater?(x=w563, y=4500.0 ("Arm Angle to Turn to")) -> (0:w560:bool)
            n281 = Greater?(x=w564, y=50.0 ("Arm Angle to Turn to")) -> (0:w559:bool)
            n282 = case shown="False" w565 {
              frame False {
              }
              frame True {
                n283 = global write "Robot Global Data.vi" "Lift Height to rase to (in)"(67.0 ("Arm Angle to Turn to")) -> ()
                n284 = global write "Robot Global Data.vi" "Arm Angle to Turn to"(7000.0 ("Arm Angle to Turn to")) -> ()
              }
            }
            n285 = And(x=w560, y=w559) -> (x .and. y?=w555:bool)
            n286 = Less?(x=w554, y=-50.0) -> (x < y?=w556:bool)
            n287 = And(x=w555, y=w556) -> (x .and. y?=w557:bool)
            n288 = case shown="True" w557 {
              frame False {
              }
              frame True {
                n289 = global write "Robot Global Data.vi" "Intake Speed Override"(-0.3 ("Arm Angle to Turn to")) -> ()
              }
            }
          }
        }
      }
      frame 10 {
        n290 = case shown="1" w575 {
          tunnel: [FALSE TRUE] -> w574
          tunnel: [0.0 w581] -> w573
          tunnel: w572 -> [_ w582]
          tunnel: [_ w579] -> w571
          tunnel: [_ w578] -> w570
          frame -1, Default {
          }
          frame 1 {
            n291 = global read "Robot Global Data.vi" "Arm Encoder New Reading"() -> (w593:dbl)
            n292 = global read "Robot Global Data.vi" "Lift Encoder Distance"() -> (w594:dbl)
            n293 = Greater?(x=w593, y=4500.0 ("Arm Angle to Turn to")) -> (0:w590:bool)
            n294 = Greater?(x=w594, y=55.0 ("Arm Angle to Turn to")) -> (0:w589:bool)
            n295 = And(x=w590, y=w589) -> (x .and. y?=w585:bool)
            n296 = Less?(x=w582, y=-395.0) -> (x < y?=w586:bool)
            n297 = Less?(x=w582, y=-350.0) -> (x < y?=w595:bool)
            n298 = And(x=w585, y=w586) -> (x .and. y?=w587:bool)
            n299 = Less?(x=w582, y=-285.0) -> (x < y?=w597:bool)
            n300 = case shown="True" w595 {
              tunnel: [_ T1 {"proportional gain (Kc)"=0.03, "integral time (Ti, min)"=0.0, "derivative time (Td, min)"=0.0} ("t")] -> w578
              tunnel: [_ TRUE] -> w579
              frame False {
              }
              frame True {
              }
            }
            n301 = case shown="True" w587 {
              frame False {
              }
              frame True {
                n302 = global write "Robot Global Data.vi" "Intake Speed Override"(-0.5 ("Arm Angle to Turn to")) -> ()
              }
            }
            n303 = case shown="False" w597 {
              tunnel: [w605 -15.0] -> w581
              tunnel: w582 -> [w604 _]
              frame False {
                n304 = Less?(x=w604, y=-115.0) -> (x < y?=w607:bool)
                n305 = case shown="True" w607 {
                  tunnel: [0.0 90.0] -> w605
                  frame False {
                  }
                  frame True {
                  }
                }
              }
              frame True {
              }
            }
            n306 = Less?(x=w582, y=-250.0) -> (x < y?=w583:bool)
            n307 = case shown="True" w583 {
              frame False {
              }
              frame True {
                n308 = global write "Robot Global Data.vi" "Lift Height to rase to (in)"(67.0 ("Arm Angle to Turn to")) -> ()
                n309 = global write "Robot Global Data.vi" "Arm Angle to Turn to"(7000.0 ("Arm Angle to Turn to")) -> ()
              }
            }
          }
        }
      }
      frame 11 {
        n310 = case shown="2" w614 {
          tunnel: [FALSE TRUE TRUE] -> w613
          tunnel: [0.0 w617 w632] -> w612
          tunnel: w611 -> [_ w618 w633]
          frame -1, Default {
          }
          frame 1 {
            n311 = Less?(x=w618, y=-300.0) -> (x < y?=w620:bool)
            n312 = case shown="False" w620 {
              tunnel: [w623 270.0] -> w617
              tunnel: w618 -> [w622 _]
              frame False {
                n313 = Less?(x=w622, y=-100.0) -> (x < y?=w625:bool)
                n314 = case shown="True" w625 {
                  tunnel: [0.0 90.0] -> w623
                  frame False {
                  }
                  frame True {
                  }
                }
              }
              frame True {
                n315 = global write "Robot Global Data.vi" "Lift Height to rase to (in)"(20.0 ("Arm Angle to Turn to")) -> ()
                n316 = global write "Robot Global Data.vi" "Arm Angle to Turn to"(7000.0 ("Arm Angle to Turn to")) -> ()
              }
            }
          }
          frame 2 {
            n317 = Greater?(x=w633, y=70.0) -> (0:w636:bool)
            n318 = case shown="True" w636 {
              frame False {
              }
              frame True {
                n319 = global write "Robot Global Data.vi" "Intake Speed Override"(1.0 ("Arm Angle to Turn to")) -> ()
                n320 = global write "Robot Global Data.vi" "Intake Pistons"(WPI_SolenoidValue."On" ("Intake Pistons")) -> ()
              }
            }
            n321 = Greater?(x=w633, y=100.0) -> (0:w634:bool)
            n322 = case shown="False" w634 {
              tunnel: [w641 -270.0] -> w632
              tunnel: w633 -> [w638 _]
              frame False {
                n323 = Greater?(x=w638, y=50.0) -> (0:w639:bool)
                n324 = case shown="False" w639 {
                  tunnel: [w645 -180.0] -> w641
                  tunnel: w638 -> [w644 _]
                  frame False {
                    n325 = Greater?(x=w644, y=25.0) -> (0:w642:bool)
                    n326 = case shown="False" w642 {
                      tunnel: w644 -> [w648 _]
                      tunnel: [w646 -90.0] -> w645
                      frame False {
                        n327 = Greater?(x=w648, y=8.5) -> (0:w649:bool)
                        n328 = case shown="True" w649 {
                          tunnel: [0.0 -90.0] -> w646
                          frame False {
                          }
                          frame True {
                            n329 = global write "Robot Global Data.vi" "Arm Angle to Turn to"(0.0 ("Arm Angle to Turn to")) -> ()
                          }
                        }
                      }
                      frame True {
                        n330 = global write "Robot Global Data.vi" "Lift Height to rase to (in)"(0.0 ("Arm Angle to Turn to")) -> ()
                      }
                    }
                  }
                  frame True {
                  }
                }
              }
              frame True {
              }
            }
          }
        }
      }
      frame 12 {
        n331 = case shown="1" w664 {
          tunnel: [FALSE TRUE TRUE TRUE] -> w663
          tunnel: [0.0 w670 w684 w711] -> w662
          tunnel: w661 -> [_ w668 w678 w708]
          tunnel: [_ _ _ w707] -> w660
          tunnel: [_ _ _ w706] -> w659
          frame -1, Default {
          }
          frame 1 {
            n332 = Less?(x=w668, y=-60.0) -> (x < y?=w672:bool)
            n333 = Less?(x=w668, y=-130.0) -> (x < y?=w667:bool)
            n334 = case shown="False" w672 {
              tunnel: [0.0 90.0] -> w670
              frame False {
              }
              frame True {
              }
            }
            n335 = case shown="False" w667 {
              frame False {
              }
              frame True {
                n336 = global write "Robot Global Data.vi" "Lift Height to rase to (in)"(30.0 ("Auto Running")) -> ()
                n337 = global write "Robot Global Data.vi" "Arm Angle to Turn to"(7000.0 ("Auto Running")) -> ()
              }
            }
          }
          frame 2 {
            n338 = Greater?(x=w678, y=250.0) -> (0:w681:bool)
            n339 = Greater?(x=w678, y=185.0) -> (0:w679:bool)
            n340 = case shown="False" w679 {
              tunnel: [w688 270.0] -> w684
              tunnel: w678 -> [w685 _]
              frame False {
                n341 = Greater?(x=w685, y=107.0) -> (0:w686:bool)
                n342 = case shown="False" w686 {
                  tunnel: [w692 180.0] -> w688
                  tunnel: w685 -> [w689 _]
                  frame False {
                    n343 = Greater?(x=w689, y=86.0) -> (0:w690:bool)
                    n344 = case shown="False" w690 {
                      tunnel: w689 -> [w695 _]
                      tunnel: [w693 90.0] -> w692
                      frame False {
                        n345 = Greater?(x=w695, y=5.0) -> (0:w696:bool)
                        n346 = case shown="True" w696 {
                          tunnel: [0.0 90.0] -> w693
                          frame False {
                          }
                          frame True {
                            n347 = global write "Robot Global Data.vi" "Arm Angle to Turn to"(0.0 ("Arm Angle to Turn to")) -> ()
                          }
                        }
                      }
                      frame True {
                        n348 = global write "Robot Global Data.vi" "Lift Height to rase to (in)"(0.0 ("Arm Angle to Turn to")) -> ()
                      }
                    }
                  }
                  frame True {
                  }
                }
              }
              frame True {
                n349 = global write "Robot Global Data.vi" "Intake Pistons"(WPI_SolenoidValue."On" ("Intake Pistons")) -> ()
              }
            }
            n350 = case shown="True" w681 {
              frame False {
              }
              frame True {
                n351 = global write "Robot Global Data.vi" "Intake Speed Override"(1.0 ("Arm Angle to Turn to")) -> ()
              }
            }
          }
          frame 3 {
            n352 = Less?(x=w708, y=-130.0) -> (x < y?=w723:bool)
            n353 = case shown="False" w723 {
              frame False {
              }
              frame True {
                n354 = global write "Robot Global Data.vi" "Lift Height to rase to (in)"(67.0 ("Arm Angle to Turn to")) -> ()
                n355 = global write "Robot Global Data.vi" "Arm Angle to Turn to"(7000.0 ("Arm Angle to Turn to")) -> ()
              }
            }
            n356 = global read "Robot Global Data.vi" "Arm Encoder New Reading"() -> (w719:dbl)
            n357 = global read "Robot Global Data.vi" "Lift Encoder Distance"() -> (w720:dbl)
            n358 = Less?(x=w708, y=-85.0) -> (x < y?=w712:bool)
            n359 = Greater?(x=w719, y=4750.0 ("Arm Angle to Turn to")) -> (0:w716:bool)
            n360 = Greater?(x=w720, y=50.0 ("Arm Angle to Turn to")) -> (0:w715:bool)
            n361 = case shown="False" w712 {
              tunnel: [90.0 0.0] -> w711
              frame False {
              }
              frame True {
              }
            }
            n362 = And(x=w716, y=w715) -> (x .and. y?=w714:bool)
            n363 = case shown="True" w714 {
              frame False {
              }
              frame True {
                n364 = global write "Robot Global Data.vi" "Intake Speed Override"(-0.3 ("Arm Angle to Turn to")) -> ()
              }
            }
            n365 = Less?(x=w708, y=-10.0) -> (x < y?=w709:bool)
            n366 = case shown="True" w709 {
              tunnel: [FALSE TRUE] -> w707
              tunnel: [cluster{"output high":dbl, "output low":dbl} {"output high"=0.7, "output low"=-0.7} ("s? t:f") cluster{"output high":dbl, "output low":dbl} {"output high"=0.7, "output low"=-1.0} ("s? t:f")] -> w706
              frame False {
              }
              frame True {
              }
            }
          }
        }
      }
    }
    n367 = Select(t=w22, s=w24, f="Angle Offset") -> (s? t:f=w26:dbl)
    n368 = Select(t=w18, s=w19, f="PID Gains X") -> (s? t:f=w20:T1)
    n369 = Select(t=w15, s=w14, f="Motor Output Range Y") -> (s? t:f=w16:cluster{"output high":dbl, "output low":dbl})
    n370 = call-poly <vilib>:"PID.vi"("output range"="Motor Output Range X", "PID gains"=w20, "process variable"=w29, "setpoint"=w26) -> ("output"=w33:dbl)  [unwired: 6 in, 1 out]
    n371 = call-poly <vilib>:"PID.vi"("output range"=w16, "PID gains"="PID Gains Y", "process variable"=w27, "setpoint"="Distance (in)") -> ("output"=w53:dbl)  [unwired: 6 in, 1 out]
    n372 = Negate(x=w53) -> (-x=w54:dbl)
    n373 = call-poly <vilib>:"WPI_RobotDriveArcadeDrive.vi"("Y axis value"=w54, "X axis value"=w33, "RobotDriveDevRef"=w55) -> ("RobotDriveDevRef"=w49:T2)  [unwired: 6 in, 2 out]
    n374 = And(x=w46, y=w45) -> (x .and. y?=w41:bool)
    n375 = Or(x=w40, y=w41) -> (x .or. y?=w42:bool)
  }
  "RobotDriveDevRef Out" <- w4
